vi "Configure Digital Filters.vi"(0 "VISA resource name":refnum<visa-resource-name>, 1 "Enable Median Filter (F: Disable)":bool, 2 "Median Filter Rank (1)":u16(ring)=1 items=["1"=1, "2"=2, "3"=3, "4"=4, "5"=5], 5 "Digital Filter Count (10)":i32=10, 7 "Digital Filter Type (0: Repeating)":u16(ring) items=["Repeating", "Moving"], 9 "Enable Digital Filter (0: Disable)":u16(ring) items=["Disable", "Enable", "Advanced"], 11 "error in (no error)":errorcluster, 12 "Digital Filter Noise Tolerance (0%)":dbl) -> (4 "VISA resource name out":refnum<visa-resource-name>, 15 "error out":errorcluster)   [LabVIEW 2024, in "Keithley 648X Series.lvlib"]
doc: "Configures the two digital filters (median and average). The output of the median filter is pushed into the average (digital) buffer."
uses:
  <instrlib>/Keithley 648X Series/Keithley 648X Series.lvlib
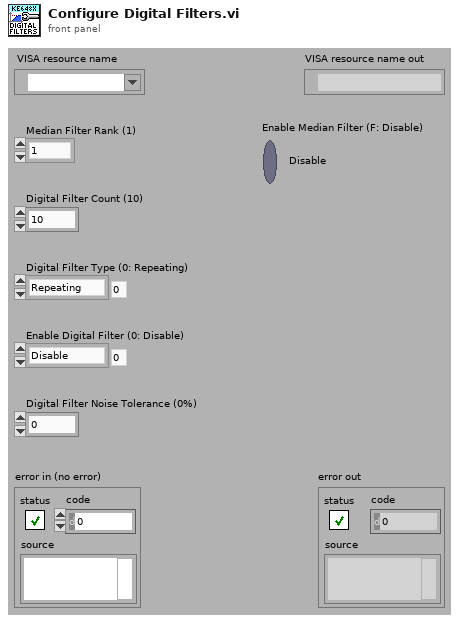
[diagram p1: front panel]
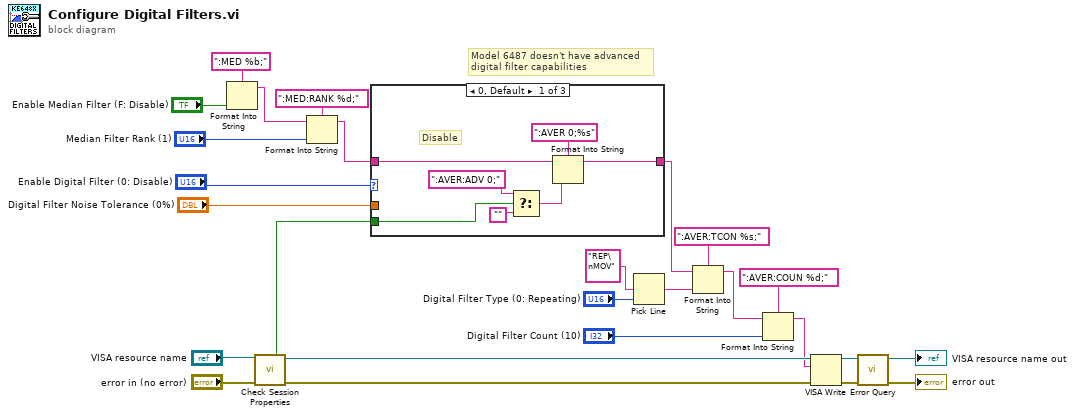
[diagram p0: block diagram]
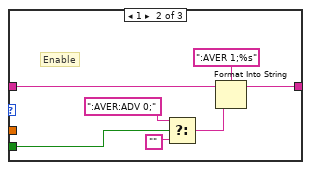
[diagram p2: hidden frame]
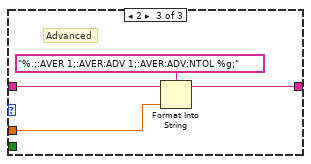
[diagram p3: hidden frame]
diagram:
  # "Model 6487 doesn't have advanced\ndigital filter capabilities"
  n1 = Format Into String(format string=":MED %b;", "Enable Median Filter (F: Disable)") -> (resulting string=w20:string)  [unwired: 2 in, 1 out]
  n2 = call <instrlib>:"Check Session Properties.vi"("VISA resource name"="VISA resource name", "error in (no error)"="error in (no error)") -> ("Model 6485"=w2:bool, "VISA resource name out"=w12:refnum<visa-resource-name>, "error out"=w13:errorcluster)  [unwired: 10 in, 1 out]
  n3 = Format Into String(format string=":MED:RANK %d;", initial string=w20, "Median Filter Rank (1)") -> (resulting string=w17:string)  [unwired: 1 in, 1 out]
  n4 = case shown="0, Default" "Enable Digital Filter (0: Disable)" {
    tunnel: w17 -> [w31 w35 w43]
    tunnel: w2 -> [w28 w38 _]
    tunnel: [w27 w34 w42] -> w10
    tunnel: "Digital Filter Noise Tolerance (0%)" -> [_ _ w41]
    frame 0, Default {
      # "Disable"
      n5 = Select(t=":AVER:ADV 0;", s=w28, f="") -> (s? t:f=w33:string)
      n6 = Format Into String(format string=":AVER 0;%s", initial string=w31, w33) -> (resulting string=w27:string)  [unwired: 1 in, 1 out]
    }
    frame 1 {
      # "Enable"
      n7 = Select(t=":AVER:ADV 0;", s=w38, f="") -> (s? t:f=w36:string)
      n8 = Format Into String(format string=":AVER 1;%s", initial string=w35, w36) -> (resulting string=w34:string)  [unwired: 1 in, 1 out]
    }
    frame 2 {
      # "Advanced"
      n9 = Format Into String(format string="%.;:AVER 1;:AVER:ADV 1;:AVER:ADV:NTOL %g;", initial string=w43, w41) -> (resulting string=w42:string)  [unwired: 1 in, 1 out]
    }
  }
  n10 = Pick Line(multi-line string="REP\nMOV", line index="Digital Filter Type (0: Repeating)") -> (output string=w7:string)  [unwired: 1 in]
  n11 = Format Into String(format string=":AVER:TCON %s;", initial string=w10, w7) -> (resulting string=w5:string)  [unwired: 1 in, 1 out]
  n12 = Format Into String(format string=":AVER:COUN %d;", initial string=w5, "Digital Filter Count (10)") -> (resulting string=w1:string)  [unwired: 1 in, 1 out]
  n13 = VISA Write(VISA resource name=w12, write buffer=w1, error in (no error)=w13) -> (VISA resource name out=w24:refnum<visa-resource-name>, error out=w23:errorcluster)  [unwired: 1 out]
  n14 = call <instrlib>:"Error Query.vi"("error in (no error)"=w23, "VISA resource name"=w24) -> ("error out"=→"error out":errorcluster, "VISA resource name out"=→"VISA resource name out":refnum<visa-resource-name>)  [unwired: 6 in, 2 out]
